vi "Alarm Loop.vi"(1 "Loop ID":T1, 11 "error out":errorcluster) -> ()   [LabVIEW 2011]
uses:
  Loop ID.ctl
  <vilib>/sound2/lvsound2.llb/Sound Output Task ID.ctl
  <vilib>/sound2/lvsound2.llb/Sampling Mode.ctl
  <vilib>/sound2/lvsound2.llb/Sound Data Format.ctl
  emi Lib/Basic/0 - General/Error/Private/_emi_Filter type.ctl
  emi Lib/Basic/0 - General/Error/Private/emi_Error Filter Array.vi
  emi Lib/System 01/0 - General/App/Loop control 2/Private/_emi_ SMLoop start condition.vi
  emi Lib/System 01/0 - General/App/Loop control 2/Private/_emi_ SMLoop Error Check.vi
  emi Lib/Basic/0 - General/Error/emi_Is Error.vi
  emi Lib/System 01/0 - General/App/Loop control 2/Private/_emi_SMLoop Register new.vi
  emi Lib/System 01/0 - General/S&E reporting/emi_Send S&E Error message.vi
  emi Lib/Basic/0 - General/Error/emi_ Is Error state.vi
  emi Lib/System 01/0 - General/emi_Read System ID.vi
  emi Lib/System 01/0 - General/App/Loop control/Private/_emi_GFV Loop Linking.vi
  emi Lib/System 01/0 - General/App/Loop control/Private/_emi_GFV Loop Enable.vi
  emi Lib/System 01/0 - General/App/Loop control 2/Private/_emi_ SMLoop Restart.vi
  emi Lib/System 01/0 - General/App/Private/_emi_GFV App Close.vi
  emi Lib/System 01/0 - General/App/Loop control 2/Private/_emi_ SMLoop Restart Counter.vi
  emi Lib/System 01/0 - General/App/Loop control/Private/_emi_GFV Loop Running.vi
  emi Lib/System 01/0 - General/Private/_emi_GFV System ID.vi
  emi Lib/System 01/0 - General/S&E reporting/Private/_emi_S&E Q Generator.vi
  <vilib>/Utility/error.llb/Clear Errors.vi
  emi Lib/System 01/0 - General/App/Loop control/Private/_emi_GFV stop a loop so it can reset.vi
  <vilib>/sound2/lvsound2.llb/Sound Output Set Volume (Single).vi
  <vilib>/sound2/lvsound2.llb/Sound Output Write (DBL Single).vi
  <vilib>/measure/NI_MABase.lvlib
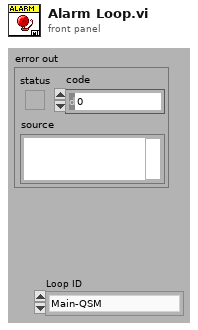
[diagram p1: front panel]
types:
  T1 = typedef "Loop ID.ctl" = enum16{"Main-QSM", "Main-Dialog", "Main-Ind Upd", "Main-Graph Upd", "Main-Debug", "Main-DebugW1", "Main-DebugW2", "Main-SE Handler", "Interface-PCP", "Interface-CANbus", "Interface-Modem", "Var Handling-Beat", "Var Handling-From PCP", "Var Handling-File storage", "Var Handling-From Simulator", "GUI-GrphW Mast", "GUI-GrphW Slav", "SIM-Tool W1", "SIM-Tool W2", "Alm-Sound", "LEIN-motor", "Tool data gatherer Qer", "Tool Data LEIN STAT2 dekoder", "Indicator Value Update", "Tool STAT2 dedicated reader", "Tool ID handler", "Detail View L1", "Detail View L2", "Main display enable view", "Sequence runner", "Voltage setpoint", "Resistance setpoint", "Stroker Wizard L1", "Stroker Wizard L2", "Alarm Handling", "Annotations Tip Strip", "Magna Interface", "Modem Status", "Var Handling - Modem Status", "Power interface detector"}
  T2 = typedef "_emi_Filter type.ctl" = enum16{"Error&Warning", "Warning", "Error"}
  T3 = typedef "_emi_ SMLoop sates.ctl" = enum16{"Init", "Standby", "Start", "Normal Operation", "Stop", "Error Handling", "End", "Post"}
  T4 = typedef "Sound Output Task ID.ctl" = u32
  T5 = cluster{"Placeholder":bool, "Sound":waveform(dbl), "task ID":T4}
  T6 = typedef "Sampling Mode.ctl" = i32
  T7 = typedef "Sound Data Format.ctl" = cluster{"sample rate (S/s)":dbl, "number of channels":i32, "bits per sample":i32}
  T8 = typedef "Options  All pages and custom.ctl" = cluster{"P 1 (App)":T9, "P 2":T10, "P 3":T11, "P 4":T14, "P 5":T19, "P 6 (Err)":T20, "P 7 (Expert)":T21, "P 8 (Depth)":T23, "C 1":T24, "C 2":T25}
  T9 = typedef "Options Page 1 (App).ctl" = cluster{"Result files":path, "PCP Interface":string, "Tractor/Stroker Interface":string, "Tractor Interface":string, "Modem Status Interface":string, "Audible Alarm":bool, "Force alarm on Technical":bool, "Force alarm on HH":bool, "Force alarm on LL":bool, "Force alarm on H":bool, "Force alarm on L":bool}
  T10 = typedef "Options Page 2.ctl" = cluster{"Solenoid & Relay latching time":u16, "Tractor relay 1":dbl, "Tractor relay 2":dbl, "Tractor Solenoid limit":dbl}
  T11 = typedef "Options Page 3.ctl" = cluster{"Min resistance":dbl, "Max resistance":dbl, "Head voltage range":T12, "Max voltage jump":dbl, "Maximum resistance change":dbl, "Start Telemetry Voltage":dbl, "Start Telemetry Timeout":dbl, "Start Motor Voltage":dbl, "Stop Motor Voltage":dbl, "Pass Mode Warning Voltage":dbl, "Relay Switch Voltage":dbl, "Relay Status Loss Voltage":dbl, "Samples to average":i32, "PSU type DO NOT USE":T13, "Magna OVP":dbl, "Magna Current Limit":dbl}
  T12 = typedef "PCP type List.ctl" = enum16{"0 - 350V", "0 - 450V", "0 - 600V"}
  T13 = typedef "PSU Type.ctl" = enum16{"Unipower", "Magna 8.3A", "Magna 12A", "None"}
  T14 = typedef "Options Page 4.ctl" = cluster{"Solenoid & Relay latching time":u16, "Stroker relay 1":dbl, "Stroker Relay 2":dbl, "Stroker Solenoid limit":dbl, "Force det.":T15, "Stroke force lim.":dbl, "Anchor Enabled Pressure":dbl, "Tacometer puls":dbl, "Default anchor behavior":T16, "Default stroker behavior":T17, "Default stroker force limit (tonne)":dbl, "Slips Size":T18}
  T15 = typedef "Stroke force selector.ctl" = enum16{"Stroke in = node 1", "Strok out = node 1"}
  T16 = typedef "Default anchor behavior.ctl" = enum16{"Do nothing", "Set Anchor", "Release Anchor"}
  T17 = typedef "Default stroker behavior.ctl" = enum16{"Do nothing", "Stop", "Go Out", "Go In"}
  T18 = typedef "Slips Type Radio.ctl" = enum32{"No Selection", "338 MRS", "3,9 MRS"}
  T19 = typedef "Options Page 5.ctl" = cluster{"Solenoid & Relay latching time":u16, "Driller relay 1":dbl, "Driller Relay 2":dbl, "Driller  Solenoid limit":dbl}
  T20 = typedef "Options Page 6 (Err).ctl" = cluster{"Error and event files":path}
  T21 = typedef "Options Page 7 (Expert).ctl" = cluster{"Show Debug":bool, "Log debug messages":bool, "Additional debug messages":bool, "Start Beagle with Simulator data":bool, "Workshop mode":bool, "Modem baud":u16, "enumCANCOM":bool, "Modem sim":T22, "Telemetry Timeout Disable":i32, "Buffer size":i32, "Upd regular data":bool, "Cable comp":cluster{"VMOD1 Voltage(V)":dbl, "VMOD2 Voltage(V)":dbl}}
  T22 = typedef "Modem simulation setup.ctl" = cluster{"Modem dealay sim":bool, "Sim baud Tx":u16, "Bit Error fraction Tx":dbl, "Sim baud Rx":u16, "Bit Error fraction Rx":dbl}
  T23 = typedef "Options Page 8 (Depth).ctl" = cluster{"Winch Spool Circumference":dbl, "Winch Pulses per Revolution":dbl, "Current Depth":dbl}
  T24 = typedef "Options Custom 1.ctl" = cluster{"Depth Updated":bool, "Depth Offset":dbl}
  T25 = typedef "Options Custom 2.ctl" = cluster{"Placeholder":bool}
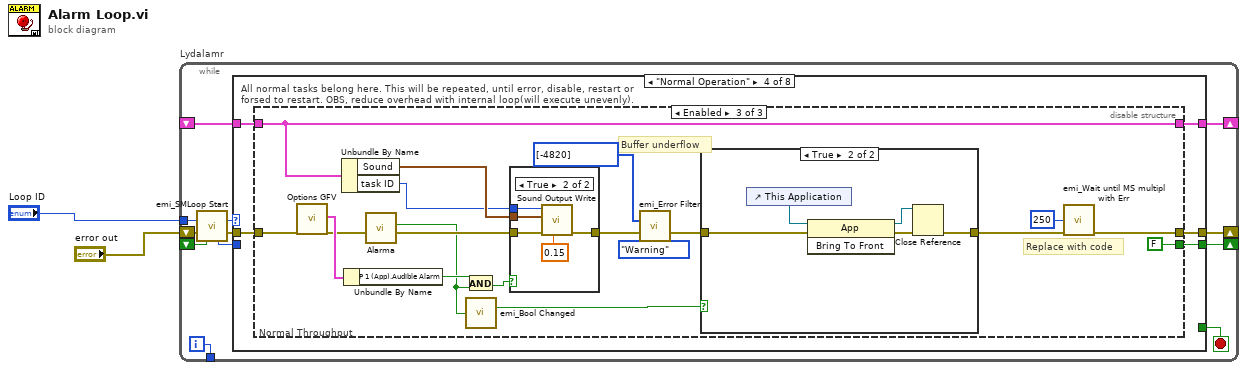
[diagram p0: block diagram]
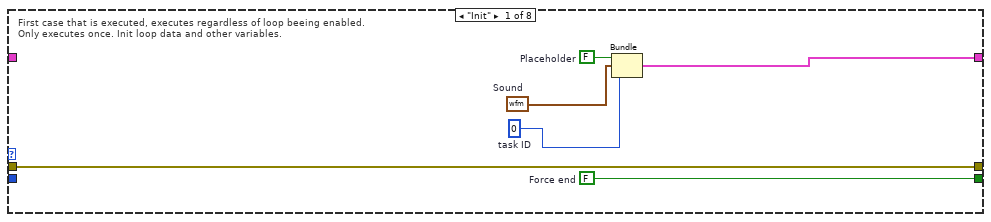
[diagram p2: hidden frame]
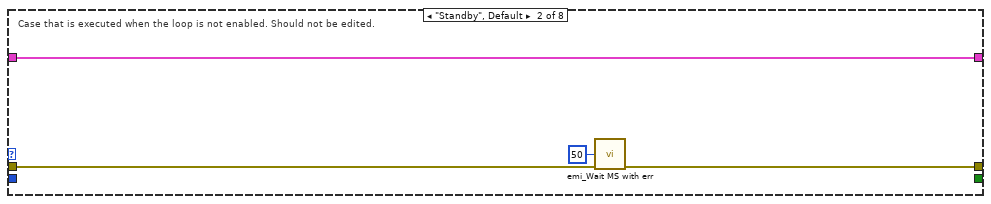
[diagram p3: hidden frame]
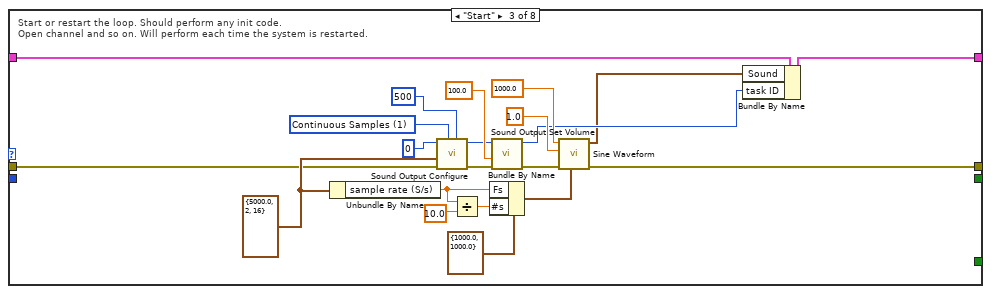
[diagram p4: hidden frame]
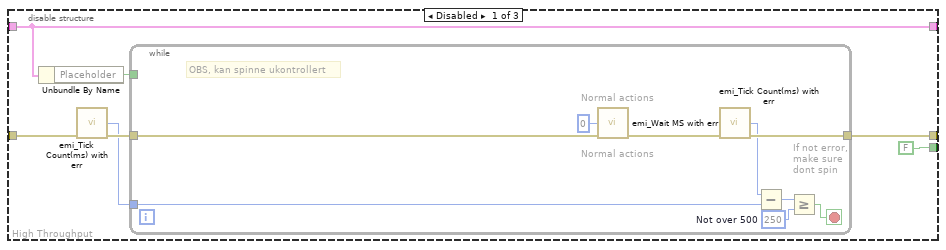
[diagram p5: hidden frame]
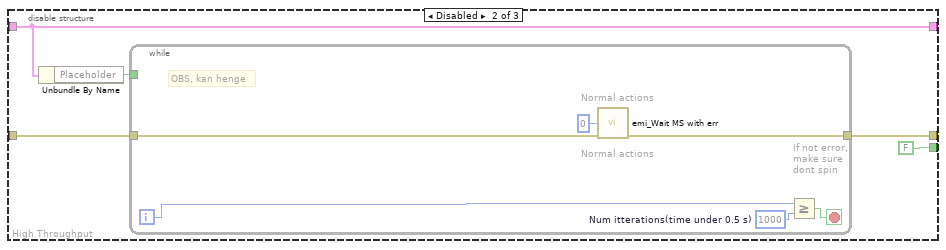
[diagram p6: hidden frame]
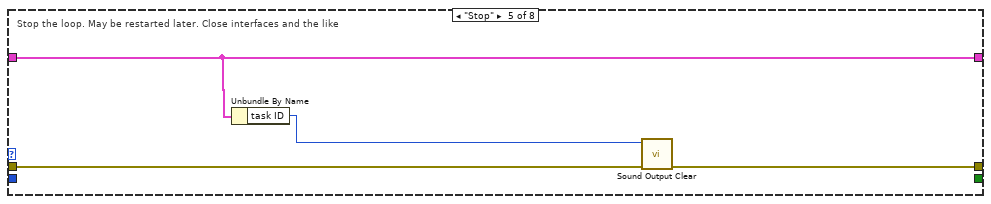
[diagram p9: hidden frame]
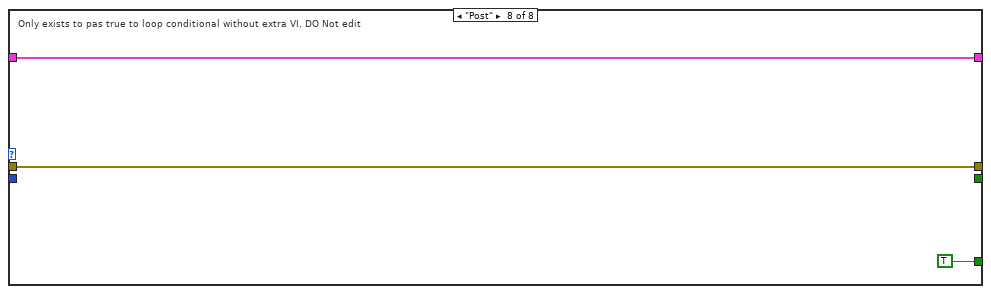
[diagram p12: hidden frame]
diagram:
  n1 = while "Lydalamr" {
    shift-right: [w14] -> _
    shift-left: _ -> [w10]
    shift-right: [w12] -> _
    shift-left: "error out" -> [w8]
    tunnel: [w11] -> _
    shift-right: [w9] -> _
    shift-left: _ -> [w5]
    tunnel: "Loop ID" -> [w3]
    i -> [w11]
    stop <- w13 stop-if-true
    n2 = call "emi_SMLoop Start.vi"("Loop ID"=w3, "error in (no error)"=w8, "Force Stop(F)"=w5) -> ("Loop command"=w6:T3, "error out"=w7:errorcluster, "Loop ID out"=w4:i32)  [unwired: 10 in]
    n3 = case shown="\"Normal Operation\"" w6 {
      tunnel: [w19 w21 w27 w48 w111 w114 w115 w118] -> w14
      tunnel: [_ _ _ _ _ _ _ TRUE] -> w13
      tunnel: w7 -> [w20 w23 w29 w50 w110 w113 w116 w119]
      tunnel: [w20 w22 w28 w49 w109 w113 w116 w119] -> w12
      tunnel: w10 -> [_ w21 w45 w47 w111 w114 w115 w118]
      tunnel: [w17 _ _ w46 _ _ _ _] -> w9
      tunnel: w4 -> [_ _ _ _ _ _ _ _]
      frame "Init" {
        w15 = T4 0  # task ID
        w16 = waveform(dbl) {"t0"=timestamp(0 s since 1904-01-01), "dt"=1.0, "Y"=[]}  # Sound
        w17 = FALSE  # Force end
        w18 = FALSE  # Placeholder
        # "First case that is executed, executes regardless of loop beeing enabled.\nOnly executes once. Init loop data and other variables."
        n4 = Bundle("Placeholder"=w18, "Sound"=w16, "task ID"=w15) -> (w19:T5)  [unwired: 1 in]
      }
      frame "Standby", Default {
        # "Case that is executed when the loop is not enabled. Should not be edited."
        n5 = call "emi_Wait MS with err.vi"("milliseconds to wait(0)"=u32 50, "error in (no error)"=w23) -> ("error out"=w22:errorcluster)  [unwired: 13 in]
      }
      frame "Start" {
        w44 = T6 1 items=["Finite Samples", "Continuous Samples"] ("sample mode")
        w34 = T7 {"sample rate (S/s)"=5000.0, "number of channels"=2, "bits per sample"=16} ("Sound Format")
        # "Start or restart the loop. Should perform any init code. \nOpen channel and so on. Will perform each time the system is restarted."
        n6 = Unbundle By Name(w34) -> ("sample rate (S/s)"=w36:dbl)
        n7 = call <vilib>:"Sound Output Configure.vi"("number of samples/ch"=500, "sample mode"=w44, "error in (no error)"=w29, "sound format"=w34, "device ID"=u32 0) -> ("error out"=w39:errorcluster, "task ID"=w41:T4)  [unwired: 5 in]
        n8 = Divide(x=w36, y=10.0) -> (x/y=w38:dbl)
        n9 = Bundle By Name(cluster=cluster{"Fs":dbl, "#s":dbl} {"Fs"=1000.0, "#s"=1000.0} ("sampling info"), "Fs"=w36, "#s"=w38) -> (w35:cluster{"Fs":dbl, "#s":dbl})
        n10 = call-poly <vilib>:"Sound Output Set Volume.vi"("error in (no error)"=w39, "volume"=100.0, "task ID"=w41) -> ("error out"=w40:errorcluster, "task ID out"=w26:T4)  [unwired: 7 in]
        n11 = call <vilib>:"Sine Waveform.vi"("sampling info"=w35, "error in (no error)"=w40, "amplitude"=1.0, "frequency"=1000.0) -> ("error out"=w28:errorcluster, "signal out"=w25:waveform(dbl))  [unwired: 6 in]
        n12 = Bundle By Name(cluster=w45, "Sound"=w25, "task ID"=w26) -> (w27:T5)
      }
      frame "Normal Operation" {
        # "All normal tasks belong here. This will be repeated, until error, disable, restart or\nforsed to restart. OBS, reduce overhead with internal loop(will execute unevenly)."
        n13 = disable-structure shown="Enabled" {
          disable-tunnel: w50 -> [w54 w67 w91]
          disable-tunnel: [w56 w70 w95] -> w49
          disable-tunnel: [w57 w71 w90] -> w48
          disable-tunnel: w47 -> [w57 w71 w90]
          disable-tunnel: [FALSE ("Force End") FALSE ("Force End") FALSE ("Force End")] -> w46
          frame Disabled {
            # "High Throughput"
            n14 = Unbundle By Name(w57) -> ("Placeholder"=w55:bool)
            n15 = call "emi_Tick Count(ms) with err.vi"("error in (no error)"=w54) -> ("millisecond timer value"=w52:u32, "error out"=w53:errorcluster)  [unwired: 13 in]
            n16 = while {
              tunnel: w53 -> [w60]
              tunnel: [w66] -> w56
              tunnel: w55 -> [_]
              tunnel: w52 -> [w65]
              stop <- w59 stop-if-true
              w62 = u32 250  # Not over 500
              # "OBS, kan spinne ukontrollert"
              # "If not error,\nmake sure \ndont spin"
              # "Normal actions"
              # "Normal actions"
              n17 = call "emi_Wait MS with err.vi"("milliseconds to wait(0)"=u32 0, "error in (no error)"=w60) -> ("error out"=w61:errorcluster)  [unwired: 13 in]
              n18 = call "emi_Tick Count(ms) with err.vi"("error in (no error)"=w61) -> ("millisecond timer value"=w64:u32, "error out"=w66:errorcluster)  [unwired: 13 in]
              n19 = Subtract(x=w64, y=w65) -> (x-y=w63:u32)
              n20 = Greater Or Equal?(x=w63, y=w62) -> (x >= y?=w59:bool)
            }
          }
          frame Disabled {
            # "High Throughput"
            n21 = Unbundle By Name(w71) -> ("Placeholder"=w69:bool)
            n22 = while {
              tunnel: [w73] -> w70
              tunnel: w69 -> [_]
              tunnel: w67 -> [w74]
              i -> [w72]
              stop <- w76 stop-if-true
              w77 = u32 1000  # Num itterations(time under 0.5 s)
              # "OBS, kan henge"
              # "If not error,\nmake sure \ndont spin"
              # "Normal actions"
              # "Normal actions"
              n23 = call "emi_Wait MS with err.vi"("milliseconds to wait(0)"=u32 0, "error in (no error)"=w74) -> ("error out"=w73:errorcluster)  [unwired: 13 in]
              n24 = Greater Or Equal?(x=w72, y=w77) -> (x >= y?=w76:bool)
            }
          }
          frame Enabled {
            # "Buffer underflow"
            # "Replace with code"
            # "Normal Throughput"
            n25 = call "Options GFV.vi"("error in (no error)"=w91) -> ("Options"=w92:T8, "error out"=w87:errorcluster)  [unwired: 16 in, 1 out]
            n26 = Unbundle By Name(w90) -> ("Sound"=w89:waveform(dbl), "task ID"=w88:T4)
            n27 = Unbundle By Name(w92) -> ("P 1 (App).Audible Alarm"=w85:bool)
            n28 = call "Alarma.vi"("error in (no error)"=w87) -> ("error out"=w86:errorcluster, "Alarma out"=w84:bool)  [unwired: 9 in]
            n29 = And(x=w85, y=w84) -> (x .and. y?=w93:bool)
            n30 = call "emi_Bool Changed.vi"("x"=w84) -> ("Rising"=w83:bool)  [unwired: 12 in, 2 out]
            n31 = case shown="True" w93 {
              tunnel: w86 -> [w103 w108]
              tunnel: [w103 w107] -> w82
              tunnel: w89 -> [_ w105]
              tunnel: w88 -> [_ w104]
              frame False {
              }
              frame True {
                n32 = call-poly <vilib>:"Sound Output Write.vi"("timeout (sec)"=0.15, "error in (no error)"=w108, "data"=w105, "task ID"=w104) -> ("error out"=w107:errorcluster)  [unwired: 6 in, 1 out]
              }
            }
            n33 = call-poly "emi_Error Filter.vi"("Error Codes"=i32[] [-4820], "error in (no error)"=w82, "Filter(Error&Warning)"=_emi_Filter_type."Warning") -> ("error out"=w80:errorcluster)  [unwired: 11 in, 1 out]
            n34 = case shown="True" w83 {
              tunnel: w80 -> [w97 w100]
              tunnel: [w97 w99] -> w81
              frame False {
              }
              frame True {
                n35 = control-ref of="This Application"() -> (w98:refnum<vi>)
                n36 = invoke class="App" method="Bring To Front"(reference=w98, error in=w100) -> (reference out=w101:refnum<vi>, error out=w102:errorcluster)  [unwired: 1 in, 1 out]
                n37 = Close Reference(reference=w101, error in (no error)=w102) -> (error out=w99:errorcluster)
              }
            }
            n38 = call "emi_Wait until MS multipl with Err.vi"("millisecond multiple(0)"=u32 250 ("milliseconds to wait(0)"), "error in (no error)"=w81) -> ("error out"=w95:errorcluster)  [unwired: 13 in]
          }
        }
      }
      frame "Stop" {
        # "Stop the loop. May be restarted later. Close interfaces and the like"
        n39 = Unbundle By Name(w111) -> ("task ID"=w112:T4)
        n40 = call <vilib>:"Sound Output Clear.vi"("error in (no error)"=w110, "task ID"=w112) -> ("error out"=w109:errorcluster)  [unwired: 9 in]
      }
      frame "Error Handling" {
        # "Loop automaticaly returns here after error is found. If error is cleared, \nLoop wil continue as normal(if was operative when error."
      }
      frame "End" {
        # "Only executes at application end has. Should performa any action the loop \nneeds to finnish. Executes only once."
      }
      frame "Post" {
        # "Only exists to pas true to loop conditional without extra VI. DO Not edit"
      }
    }
  }
